vi "HEWH Find Exact Cutout Location.vi"(8 "error in (no error)":errorcluster, 10 "Upper Most Element":T6, 11 "UEF Calculated Values Input in":T1 {"Data Indexes"."15 sec after Draw Index" format="%#.2f"; "Data Indexes"."15 sec after Draw Timestamp" format="%#.2f"; "Data Indexes"."Test Start Timestamp" format="%.2f"; "Data Indexes"."Test End Timestamp" format="%.2f"; "Data Indexes"."T0 Timestamp" format="%.2f"; "Data Indexes"."Tsf Timestamp" format="%.2f"; "Data Indexes"."Tsu0 Timestamp" format="%.2f"; "Data Indexes"."Tmax1 Timestamp" format="%.2f"; "Data Indexes"."Draw Index Timestamp" format="%#.2f"; "Data Indexes"."Non-Draw Timestamp" format="%#.2f"; "Data Indexes"."Heating Timestamp" format="%#.2f"; "Data Indexes"."Start Energy (BTU-Gas)" format="%.6f"; "Data Indexes"."Start Watt Hours" format="%.6f"; "Static Data"."V - Volume of Wh (True)" format="%.5f"; "Static Data"."T-Ambinet Nominal (°F)" format="%.5f"; "Static Data"."T-Inlet Setpoint (°F)" format="%.5f"; "Static Data"."T-Wh Setpoint (°F)" format="%.5f"; "Sampled Data"."Qe (Wh)" format="%.5f"; "Sampled Data"."Tau stby2 (hr)" format="%.5f"; "Sampled Data"."Tastby2 (°F)" format="%.5f"; "Sampled Data"."Qf (BTU)" format="%.5f"; "Sampled Data"."Qe (BTU)" format="%.5f"; "Sampled Data"."Tmax1 (°F)" format="%.5f"; "Sampled Data"."T0 (°F)" format="%.5f"; "Sampled Data"."Qr (BTU)" format="%.5f"; "Sampled Data"."T 24(°F)" format="%.5f"; "Sampled Data"."T astby(°F)" format="%.5f"; "Sampled Data"."T tstby(°F)" format="%.5f"; "Sampled Data"."T su0(°F)" format="%.5f"; "Sampled Data"."T suf(°F)" format="%.5f"; "Sampled Data"."Tau stby_1 (hr)" format="%.5f"; "Sampled Data"."Qsuf (BTU)" format="%.5f"; "Sampled Data"."Qsu0 (BTU)" format="%.5f"; "Calculated Values"."Draw Bonus Volume (gal)" format="%.6f"; "Calculated Values"."Adjustment Factor" format="%.6f"; "Calculated Values"."T*avg_del(n-1)" format="%.6f"; "Calculated Values"."T*min(n-1)" format="%.6f"; "Calculated Values"."T*avg_del(n)" format="%.6f"; "Calculated Values"."Vn" format="%.6f"; "Calculated Values"."Qdm (BTU)" format="%.6f"; "Calculated Values"."QHWD (BTU)" format="%.6f"; "Calculated Values"."QHW (BTU)" format="%.6f"; "Calculated Values"."UEF" format="%.6f"; "Calculated Values"."QHW67 (BTU)" format="%.6f"; "Calculated Values"."Qda (BTU)" format="%.6f"; "Calculated Values"."Qd (BTU)" format="%.6f"; "Calculated Values"."Q (BTU)" format="%.6f"; "Calculated Values"."UA (BTU/(hr*F))" format="%.6f"; "Calculated Values"."Qhr (BTU/hr)" format="%.6f"; "Calculated Values"."Qstby (BTU)" format="%.6f"; "Calculated Values"."nu_r" format="%.6f"; "Calculated Values"."CpUEF (BTU/(lb*F))" format="%.6f"; "Calculated Values"."rho_nu (lb/gal)" format="%.6f"; "Calculated Values"."V1- Vol (Gal)" format="%.6f"; "Calculated Values"."M cluster mass removed (lb)" format="%.6f"; "Calculated Values"."Cp theoretical (BTU/(lbm °F))" format="%.6f"; "Calculated Values"."Tin1 - Mean Inlet 1st Cluster (°F)" format="%.6f"; "Calculated Values"."Tdel1-Mean Outlet 1st Cluster(°F)" format="%.6f"; "Calculated Values"."Cp 24 (BTU/(lb*F))" format="%.6f"; "Calculated Values"."Cp standby (BTU/(lb*F))" format="%.6f"; "Calculated Values"."Cp2 (BTU/(lb*F))" format="%.6f"; "Calculated Values"."Cp1 (BTU/(lb*F))" format="%.6f"; "Calculated Values"."rho 24 (lb/gal)" format="%.6f"; "Calculated Values"."rho standby (lb/gal)" format="%.6f"; "Calculated Values"."rho 2 (lb/gal)" format="%.6f"; "Calculated Values"."Density of cold water All (lbm/gal)" format="%#.3g"; "Calculated Values"."CpHW (BTU/(lbm °F))" format="%#.3g"; "Calculated Values"."Density of hot water All (lbm/gal)" format="%#.3g"; "Calculated Values"."Mass of water All (lbm)" format="%#.3f"}) -> (0 "error out":errorcluster, 2 "Cut Out Location":dbl, 3 "UEF Calculated Values Input in 2":T1 {"Data Indexes"."15 sec after Draw Index" format="%#.2f"; "Data Indexes"."15 sec after Draw Timestamp" format="%#.2f"; "Data Indexes"."Test Start Timestamp" format="%.2f"; "Data Indexes"."Test End Timestamp" format="%.2f"; "Data Indexes"."T0 Timestamp" format="%.2f"; "Data Indexes"."Tsf Timestamp" format="%.2f"; "Data Indexes"."Tsu0 Timestamp" format="%.2f"; "Data Indexes"."Tmax1 Timestamp" format="%.2f"; "Data Indexes"."Draw Index Timestamp" format="%#.2f"; "Data Indexes"."Non-Draw Timestamp" format="%#.2f"; "Data Indexes"."Heating Timestamp" format="%#.2f"; "Data Indexes"."Start Energy (BTU-Gas)" format="%.6f"; "Data Indexes"."Start Watt Hours" format="%.6f"; "Static Data"."V - Volume of Wh (True)" format="%.5f"; "Static Data"."T-Ambinet Nominal (°F)" format="%.5f"; "Static Data"."T-Inlet Setpoint (°F)" format="%.5f"; "Static Data"."T-Wh Setpoint (°F)" format="%.5f"; "Sampled Data"."Qe (Wh)" format="%.5f"; "Sampled Data"."Tau stby2 (hr)" format="%.5f"; "Sampled Data"."Tastby2 (°F)" format="%.5f"; "Sampled Data"."Qf (BTU)" format="%.5f"; "Sampled Data"."Qe (BTU)" format="%.5f"; "Sampled Data"."Tmax1 (°F)" format="%.5f"; "Sampled Data"."T0 (°F)" format="%.5f"; "Sampled Data"."Qr (BTU)" format="%.5f"; "Sampled Data"."T 24(°F)" format="%.5f"; "Sampled Data"."T astby(°F)" format="%.5f"; "Sampled Data"."T tstby(°F)" format="%.5f"; "Sampled Data"."T su0(°F)" format="%.5f"; "Sampled Data"."T suf(°F)" format="%.5f"; "Sampled Data"."Tau stby_1 (hr)" format="%.5f"; "Sampled Data"."Qsuf (BTU)" format="%.5f"; "Sampled Data"."Qsu0 (BTU)" format="%.5f"; "Calculated Values"."Draw Bonus Volume (gal)" format="%.6f"; "Calculated Values"."Adjustment Factor" format="%.6f"; "Calculated Values"."T*avg_del(n-1)" format="%.6f"; "Calculated Values"."T*min(n-1)" format="%.6f"; "Calculated Values"."T*avg_del(n)" format="%.6f"; "Calculated Values"."Vn" format="%.6f"; "Calculated Values"."Qdm (BTU)" format="%.6f"; "Calculated Values"."QHWD (BTU)" format="%.6f"; "Calculated Values"."QHW (BTU)" format="%.6f"; "Calculated Values"."UEF" format="%.6f"; "Calculated Values"."QHW67 (BTU)" format="%.6f"; "Calculated Values"."Qda (BTU)" format="%.6f"; "Calculated Values"."Qd (BTU)" format="%.6f"; "Calculated Values"."Q (BTU)" format="%.6f"; "Calculated Values"."UA (BTU/(hr*F))" format="%.6f"; "Calculated Values"."Qhr (BTU/hr)" format="%.6f"; "Calculated Values"."Qstby (BTU)" format="%.6f"; "Calculated Values"."nu_r" format="%.6f"; "Calculated Values"."CpUEF (BTU/(lb*F))" format="%.6f"; "Calculated Values"."rho_nu (lb/gal)" format="%.6f"; "Calculated Values"."V1- Vol (Gal)" format="%.6f"; "Calculated Values"."M cluster mass removed (lb)" format="%.6f"; "Calculated Values"."Cp theoretical (BTU/(lbm °F))" format="%.6f"; "Calculated Values"."Tin1 - Mean Inlet 1st Cluster (°F)" format="%.6f"; "Calculated Values"."Tdel1-Mean Outlet 1st Cluster(°F)" format="%.6f"; "Calculated Values"."Cp 24 (BTU/(lb*F))" format="%.6f"; "Calculated Values"."Cp standby (BTU/(lb*F))" format="%.6f"; "Calculated Values"."Cp2 (BTU/(lb*F))" format="%.6f"; "Calculated Values"."Cp1 (BTU/(lb*F))" format="%.6f"; "Calculated Values"."rho 24 (lb/gal)" format="%.6f"; "Calculated Values"."rho standby (lb/gal)" format="%.6f"; "Calculated Values"."rho 2 (lb/gal)" format="%.6f"; "Calculated Values"."Density of cold water All (lbm/gal)" format="%#.3g"; "Calculated Values"."CpHW (BTU/(lbm °F))" format="%#.3g"; "Calculated Values"."Density of hot water All (lbm/gal)" format="%#.3g"; "Calculated Values"."Mass of water All (lbm)" format="%#.3f"})   [LabVIEW 2023]
uses:
  Type Definitions/UEF Constants.ctl
  Type Definitions/HEWH Draw Stats.ctl
  Type Definitions/HEWH FHR Draw Type.ctl
  Type Definitions/FHR Bins.ctl
  Type Definitions/HEWH Meter Type.ctl
  Type Definitions/Upper Most Element.ctl
panel:
  # "FHR"
  # "FHR"
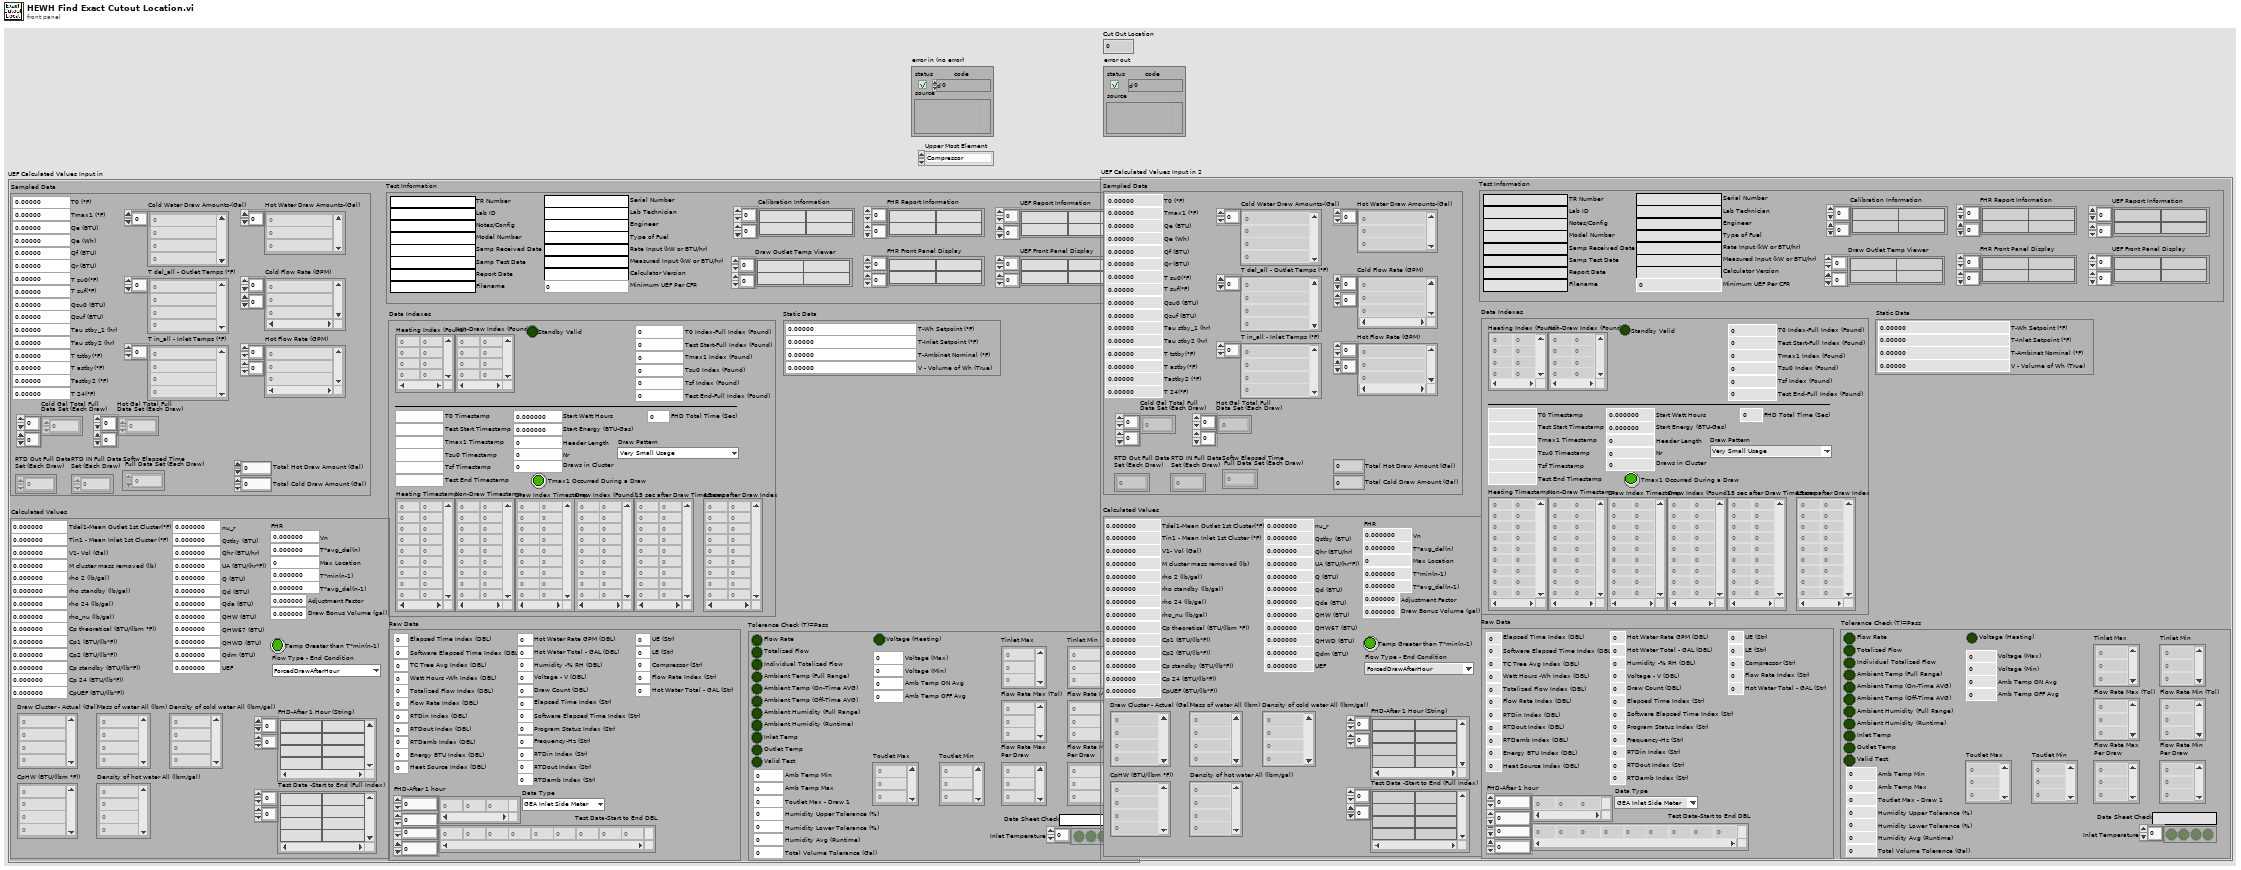
[diagram p1: front panel]
types:
  T1 = typedef "UEF Constants.ctl" = cluster{"Calculated Values":T2, "Sampled Data":cluster{"Cold Water Draw Amounts-(Gal)":dbl[], "T del_all - Outlet Temps (°F)":dbl[], "T in_all - Inlet Temps (°F)":dbl[], "Qsu0 (BTU)":dbl, "Qsuf (BTU)":dbl, "Tau stby_1 (hr)":dbl, "T suf(°F)":dbl, "T su0(°F)":dbl, "T tstby(°F)":dbl, "T astby(°F)":dbl, "T 24(°F)":dbl, "Qr (BTU)":dbl, "T0 (°F)":dbl, "Tmax1 (°F)":dbl, "Qe (BTU)":dbl, "Qf (BTU)":dbl, "Tastby2 (°F)":dbl, "RTD Out Full Data\nSet (Each Draw)":dbl[][], "RTD IN Full Data\nSet (Each Draw)":dbl[][], "Tau stby2 (hr)":dbl, "Hot Water Draw Amounts-(Gal)":dbl[], "Cold Flow Rate (GPM)":dbl[][], "Hot Flow Rate (GPM)":dbl[][], "Softw Elapsed Time\n Full Data Set (Each Draw)":dbl[][], "Cold Gal Total Full\nData Set (Each Draw)":dbl[][], "Total Hot Draw Amount (Gal) ":dbl, "Total Cold Draw Amount (Gal)":dbl, "Qe (Wh)":dbl, "Hot Gal Total Full\nData Set (Each Draw)":dbl[][]}, "Static Data":cluster{"T-Wh Setpoint (°F)":dbl, "T-Inlet Setpoint (°F)":dbl, "T-Ambinet Nominal (°F)":dbl, "V - Volume of Wh (True)":dbl}, "Data Indexes":cluster{"Test Start-Full Index (Found)":i32, "Header Length":i32, "Draw Index (Found)":i32[][], "Nr":i32, "Start Watt Hours":dbl, "Tsu0 Index (Found)":i32, "Tsf Index (Found)":i32, "Start Energy (BTU-Gas)":dbl, "Draws in Cluster":i32, "T0 Index-Full Index (Found)":i32, "Non-Draw Index (Found)":i32[][], "Tmax1 Index (Found)":i32, "Test End-Full Index (Found)":i32, "Heating Index (Found)":i32[][], "Heating Timestamp":dbl[][], "Non-Draw Timestamp":dbl[][], "Draw Index Timestamp":dbl[][], "Tmax1 Timestamp":dbl, "Tsu0 Timestamp":dbl, "Tsf Timestamp":dbl, "T0 Timestamp":dbl, "Test End Timestamp":dbl, "Test Start Timestamp":dbl, "15 sec after Draw Timestamp":dbl[][], "15 sec after Draw Index":dbl[][], "Tmax1 Occurred During a Draw":bool, "FHD Total Time (Sec)":dbl, "Draw Pattern":T4, "Standby Valid":bool}, "Raw Data":cluster{"Elapsed Time Index (DBL)":i32, "Software Elapsed Time Index (DBL)":i32, "TC Tree Avg Index (DBL)":i32, "Watt Hours -Wh Index (DBL)":i32, "Energy BTU Index (DBL)":i32, "Totalized Flow Index (DBL)":i32, "Flow Rate Index (DBL)":i32, "Program Status Index (Str)":i32, "RTDin Index (DBL)":i32, "RTDout Index (DBL)":i32, "RTDamb Index (DBL)":i32, "Test Data-Start to End DBL":dbl[][], "Data Type":T5, "Heat Source Index (DBL)":i32, "Hot Water Rate GPM (DBL)":i32, "Hot Water Total - GAL (DBL)":i32, "FHD-After 1 hour":dbl[][], "Humidity -% RH (DBL)":i32, "Voltage - V (DBL)":i32, "Draw Count (DBL)":i32, "Elapsed Time Index (Str)":i32, "Software Elapsed Time Index (Str)":i32, "Frequency-Hz (Str)":i32, "RTDin Index (Str)":i32, "RTDout Index (Str)":i32, "RTDamb Index (Str)":i32, "UE (Str)":i32, "LE (Str)":i32, "Compressor (Str)":i32, "Flow Rate Index (Str)":i32, "Hot Water Total - GAL (Str)":i32}, "Tolerance Check (T)=Pass":cluster{"Flow Rate":bool, "Totalized Flow":bool, "Ambient Temp (Full Range)":bool, "Ambient Humidity (Full Range)":bool, "Inlet Temp":bool, "Outlet Temp":bool, "Valid Test":bool, "Individual Totalized Flow":bool, "Data Sheet Check":string, "Inlet Temperature":bool[], "Tinlet Max":dbl[], "Tinlet Min":dbl[], "Flow Rate Max (Tol)":dbl[], "Flow Rate Min (Tol)":dbl[], "Amb Temp Max":dbl, "Amb Temp Min":dbl, "Toutlet Max - Draw 1":dbl, "Humidity Upper Tolerance (%)":dbl, "Total Volume Tolerance (Gal)":dbl, "Humidity Lower Tolerance (%)":dbl, "Flow Rate Max\nPer Draw":dbl[], "Flow Rate Min\nPer Draw":dbl[], "Ambient Humidity (Runtime)":bool, "Humidity Avg (Runtime)":dbl, "Ambient Temp (On-Time AVG)":bool, "Ambient Temp (Off-Time AVG)":bool, "Amb Temp OFF Avg":dbl, "Amb Temp ON Avg":dbl, "Voltage (Heating)":bool, "Voltage (Min)":dbl, "Voltage (Max)":dbl, "Toutlet Max":dbl[], "Toutlet Min":dbl[]}, "Test Information":cluster{"TR Number":string, "Lab ID":string, "Notes/Config":string, "Model Number":string, "Serial Number":string, "Lab Technician":string, "Engineer":string, "Type of Fuel":string, "Samp Received Date":string, "Samp Test Date":string, "Report Date":string, "Rate Input (kW or BTU/hr)":string, "Measured Input (kW or BTU/hr)":string, "Filename":string, "Calibration Information":string[][], "Calculator Version":string, "Minimum UEF Per CFR":dbl, "UEF Report Information":string[][], "FHR Report Information":string[][], "FHR Front Panel Display":string[][], "UEF Front Panel Display":string[][], "Draw Outlet Temp Viewer":string[][]}}
  T2 = typedef "HEWH Draw Stats.ctl" = cluster{"Draw Cluster - Actual (Gal)":dbl[], "Mass of water All (lbm)":dbl[], "Density of hot water All (lbm/gal)":dbl[], "CpHW (BTU/(lbm °F))":dbl[], "rho 2 (lb/gal)":dbl, "rho standby (lb/gal)":dbl, "rho 24 (lb/gal)":dbl, "Cp1 (BTU/(lb*F))":dbl, "Cp2 (BTU/(lb*F))":dbl, "Cp standby (BTU/(lb*F))":dbl, "Cp 24 (BTU/(lb*F))":dbl, "nu_r":dbl, "Qstby (BTU)":dbl, "Qhr (BTU/hr)":dbl, "UA (BTU/(hr*F))":dbl, "Q (BTU)":dbl, "Qd (BTU)":dbl, "Qda (BTU)":dbl, "QHW67 (BTU)":dbl, "UEF":dbl, "Tdel1-Mean Outlet 1st Cluster(°F)":dbl, "Tin1 - Mean Inlet 1st Cluster (°F)":dbl, "Cp theoretical (BTU/(lbm °F))":dbl, "M cluster mass removed (lb)":dbl, "V1- Vol (Gal)":dbl, "Test Data -Start to End (Full Index)":string[][], "rho_nu (lb/gal)":dbl, "Density of cold water All (lbm/gal)":dbl[], "CpUEF (BTU/(lb*F))":dbl, "QHW (BTU)":dbl, "QHWD (BTU)":dbl, "Qdm (BTU)":dbl, "FHD-After 1 Hour (String)":string[][], "Vn":dbl, "T*avg_del(n)":dbl, "Max Location":i32, "T*min(n-1)":dbl, "T*avg_del(n-1)":dbl, "Temp Greater than T*min(n-1)":bool, "Adjustment Factor":dbl, "Draw Bonus Volume (gal)":dbl, "Flow Type - End Condition":T3}
  T3 = typedef "HEWH FHR Draw Type.ctl" = enum16{"ForcedDrawAfterHour", "HeatingCutoffBeforeHour"}
  T4 = typedef "FHR Bins.ctl" = enum16{"Very Small Usage", "Low Usage", "Medium Usage", "High Usage", "Undefined"}
  T5 = typedef "HEWH Meter Type.ctl" = enum16{"GEA Inlet Side Meter", "GEA Outlet Side Meter", "CSA Inlet Side Meter"}
  T6 = typedef "Upper Most Element.ctl" = enum16{"Compressor", "Lower Element", "Upper Element"}
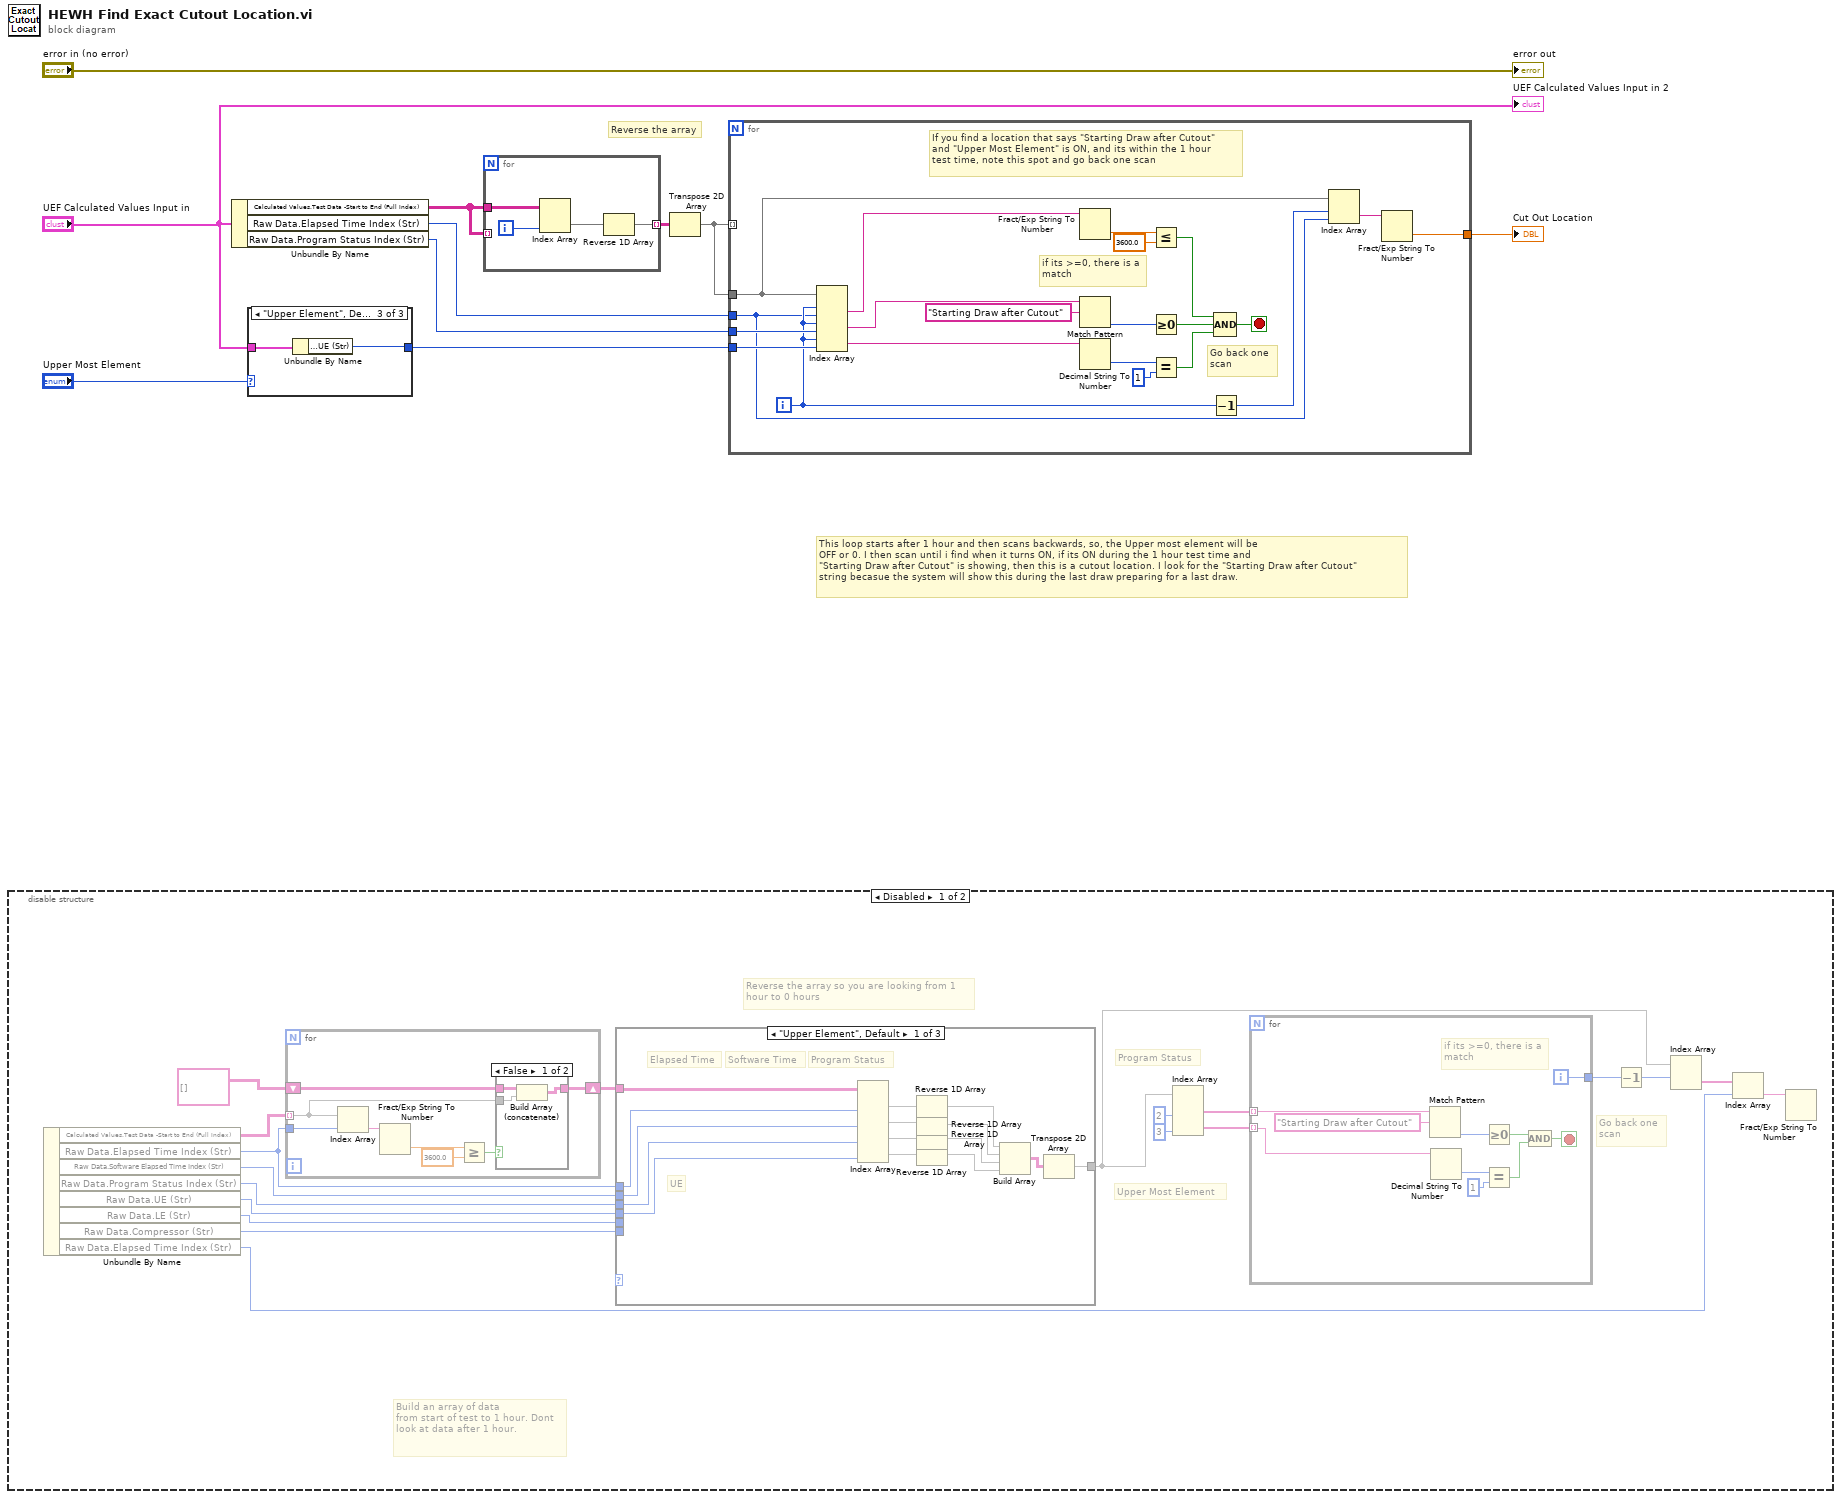
[diagram p0: block diagram]
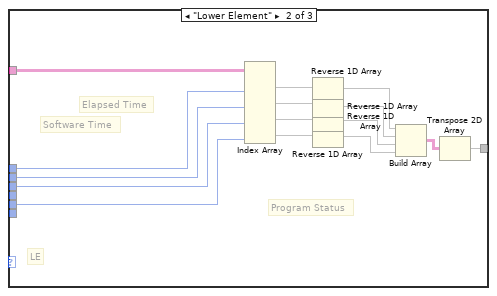
[diagram p2: hidden frame]
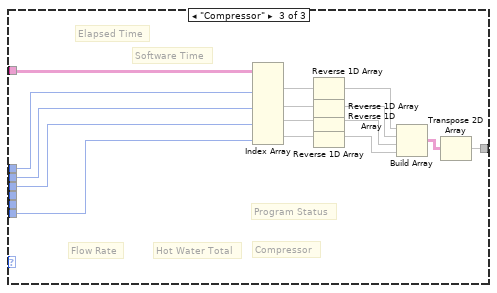
[diagram p3: hidden frame]
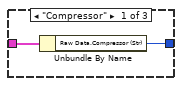
[diagram p6: hidden frame]
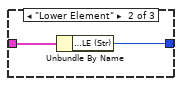
[diagram p7: hidden frame]
diagram:
  # "This loop starts after 1 hour and then scans backwards, so, the Upper most element will be \nOFF or 0. I then scan until i find when it turns ON, if its ON during the 1 hour test time and\n\"Starting Draw after Cutout\" is showing, then this is a cutout location. I look for the \"Starting Draw after Cutout\"\nstring becasue the system will show this during the last draw preparing for a last draw."
  # "Reverse the array"
  n1 = disable-structure shown="Disabled" {
    frame Disabled {
      # "Reverse the array so you are looking from 1\nhour to 0 hours"
      # "Go back one\nscan"
      # "Upper Most Element"
      # "Program Status"
      # "Build an array of data\nfrom start of test to 1 hour. Dont look at data after 1 hour."
      n2 = Unbundle By Name() -> ("Calculated Values.Test Data -Start to End (Full Index)"=w11:string[][], "Raw Data.Elapsed Time Index (Str)"=w14:i32, "Raw Data.Software Elapsed Time Index (Str)"=w20:i32, "Raw Data.Program Status Index (Str)"=w19:i32, "Raw Data.UE (Str)"=w18:i32, "Raw Data.LE (Str)"=w17:i32, "Raw Data.Compressor (Str)"=w16:i32, "Raw Data.Elapsed Time Index (Str)"=w13:i32)  [unwired: 1 in]
      n3 = for {
        tunnel: w11 -> [w86] mode=indexing
        shift-right: [w91] -> w15
        shift-left: string[][] [] -> [w92]
        tunnel: w14 -> [w85]
        n4 = Index Array(array=w86, index=w85) -> (element=w90:string)
        n5 = Fract/Exp String To Number(string=w90) -> (number=w89:dbl)  [unwired: 3 in, 1 out]
        n6 = Greater Or Equal?(x=w89, y=3600.0) -> (x >= y?=w87:bool)
        n7 = case shown="False" w87 {
          tunnel: w92 -> [w95 w96]
          tunnel: [w94 w96] -> w91
          tunnel: w86 -> [w93 _]
          frame False {
            n8 = Build Array (concatenate)(w95, w93) -> (w94:string[][])
          }
          frame True {
          }
        }
      }
      n9 = case shown="\"Upper Element\", Default" {
        selector: _ -> [_ _ _]
        tunnel: w15 -> [w53 w69 w84]
        tunnel: [w52 w59 w74] -> w26
        tunnel: w14 -> [w43 w58 w73]
        tunnel: w20 -> [w42 w57 w72]
        tunnel: w19 -> [w41 w56 w71]
        tunnel: w18 -> [w40 _ _]
        tunnel: w17 -> [_ w55 _]
        tunnel: w16 -> [_ _ w70]
        frame "Upper Element", Default {
          # "UE"
          # "Program Status"
          # "Software Time"
          # "Elapsed Time"
          n10 = Index Array(array=w53, index (col) #1=w43, index (col) #2=w42, index (col) #3=w41, index (col) #4=w40) -> (element #1=w51:string[], element #2=w49:string[], element #3=w47:string[], element #4=w45:string[])  [unwired: 4 in]
          n11 = Reverse 1D Array(array=w51) -> (reversed array=w50:string[])
          n12 = Reverse 1D Array(array=w49) -> (reversed array=w48:string[])
          n13 = Reverse 1D Array(array=w47) -> (reversed array=w46:string[])
          n14 = Reverse 1D Array(array=w45) -> (reversed array=w44:string[])
          n15 = Build Array(w50, w48, w46, w44) -> (w54:string[][])
          n16 = Transpose 2D Array(2D array=w54) -> (transposed array=w52:string[][])
        }
        frame "Lower Element" {
          # "LE"
          # "Program Status"
          # "Software Time"
          # "Elapsed Time"
          n17 = Index Array(array=w69, index (col) #1=w58, index (col) #2=w57, index (col) #3=w56, index (col) #4=w55) -> (element #1=w63:string[], element #2=w62:string[], element #3=w61:string[], element #4=w60:string[])  [unwired: 4 in]
          n18 = Reverse 1D Array(array=w63) -> (reversed array=w67:string[])
          n19 = Reverse 1D Array(array=w62) -> (reversed array=w66:string[])
          n20 = Reverse 1D Array(array=w61) -> (reversed array=w65:string[])
          n21 = Reverse 1D Array(array=w60) -> (reversed array=w64:string[])
          n22 = Build Array(w67, w66, w65, w64) -> (w68:string[][])
          n23 = Transpose 2D Array(2D array=w68) -> (transposed array=w59:string[][])
        }
        frame "Compressor" {
          # "Hot Water Total"
          # "Program Status"
          # "Flow Rate"
          # "Compressor"
          # "Software Time"
          # "Elapsed Time"
          n24 = Index Array(array=w84, index (col) #1=w73, index (col) #2=w72, index (col) #3=w71, index (col) #4=w70) -> (element #1=w78:string[], element #2=w77:string[], element #3=w76:string[], element #4=w75:string[])  [unwired: 4 in]
          n25 = Reverse 1D Array(array=w78) -> (reversed array=w82:string[])
          n26 = Reverse 1D Array(array=w77) -> (reversed array=w81:string[])
          n27 = Reverse 1D Array(array=w76) -> (reversed array=w80:string[])
          n28 = Reverse 1D Array(array=w75) -> (reversed array=w79:string[])
          n29 = Build Array(w82, w81, w80, w79) -> (w83:string[][])
          n30 = Transpose 2D Array(2D array=w83) -> (transposed array=w74:string[][])
        }
      }
      n31 = Index Array(array=w26, index (col) #1=2 ("disabled index (col)"), index (col) #2=3 ("index (col)")) -> (element #1=w12:string[], element #2=w24:string[])  [unwired: 2 in]
      n32 = for {
        tunnel: w12 -> [w39] mode=indexing
        tunnel: w24 -> [w37] mode=indexing
        tunnel: [w32] -> w25
        i -> [w32]
        stop <- w33 stop-if-true
        # "if its >=0, there is a \nmatch"
        n33 = Match Pattern(string=w39, regular expression="Starting Draw after Cutout") -> (offset past match=w31:i32)  [unwired: 1 in, 3 out]
        n34 = Decimal String To Number(string=w37) -> (number=w36:i32)  [unwired: 2 in, 1 out]
        n35 = Greater Or Equal To 0?(x=w31) -> (x >= 0?=w30:bool)
        n36 = Equal?(x=w36, y=1) -> (x = y?=w34:bool)
        n37 = Compound Arithmetic op=AND(w30, w34) -> (w33:bool)
      }
      n38 = Decrement(x=w25) -> (x-1=w27:i32)
      n39 = Index Array(array=w26, index (row)=w27) -> (element=w28:string[])  [unwired: 1 in]
      n40 = Index Array(array=w28, index=w13) -> (element=w29:string)
      n41 = Fract/Exp String To Number(string=w29) -> ()  [unwired: 3 in, 2 out]
    }
    frame Enabled {
    }
  }
  n42 = Unbundle By Name("UEF Calculated Values Input in") -> ("Calculated Values.Test Data -Start to End (Full Index)"=w2:string[][], "Raw Data.Elapsed Time Index (Str)"=w8:i32, "Raw Data.Program Status Index (Str)"=w7:i32)
  n43 = case shown="\"Upper Element\", Default" "Upper Most Element" {
    tunnel: "UEF Calculated Values Input in" -> [w98 w100 w102]
    tunnel: [w97 w99 w101] -> w4
    frame "Compressor" {
      n44 = Unbundle By Name(w98) -> ("Raw Data.Compressor (Str)"=w97:i32)
    }
    frame "Lower Element" {
      n45 = Unbundle By Name(w100) -> ("Raw Data.LE (Str)"=w99:i32)
    }
    frame "Upper Element", Default {
      n46 = Unbundle By Name(w102) -> ("Raw Data.UE (Str)"=w101:i32)
    }
  }
  n47 = for {
    tunnel: w2 -> [w106]
    tunnel: w2 -> [_] mode=indexing
    tunnel: [w103] -> w9 mode=indexing
    i -> [w105]
    n48 = Index Array(array=w106, index (col)=w105) -> (element=w104:string[])  [unwired: 1 in]
    n49 = Reverse 1D Array(array=w104) -> (reversed array=w103:string[])
  }
  n50 = Transpose 2D Array(2D array=w9) -> (transposed array=w3:string[][])
  n51 = for {
    tunnel: w3 -> [_] mode=indexing
    tunnel: w8 -> [w110]
    tunnel: w7 -> [w127]
    tunnel: w4 -> [w126]
    tunnel: w3 -> [w112]
    tunnel: [w108] -> w1
    i -> [w113]
    stop <- w107 stop-if-true
    # "Go back one\nscan"
    # "If you find a location that says \"Starting Draw after Cutout\"\nand \"Upper Most Element\" is ON, and its within the 1 hour\ntest time, note this spot and go back one scan"
    # "if its >=0, there is a \nmatch"
    n52 = Index Array(array=w112, index (row) #1=w113, index (col) #1=w110, index (row) #2=w113, index (col) #2=w127, index (row) #3=w113, index (col) #3=w126) -> (element #1=w115:string, element #2=w119:string, element #3=w118:string)
    n53 = Fract/Exp String To Number(string=w115) -> (number=w116:dbl)  [unwired: 3 in, 1 out]
    n54 = Match Pattern(string=w119, regular expression="Starting Draw after Cutout") -> (offset past match=w123:i32)  [unwired: 1 in, 3 out]
    n55 = Decimal String To Number(string=w118) -> (number=w125:i32)  [unwired: 2 in, 1 out]
    n56 = Less Or Equal?(x=w116, y=3600.0) -> (x <= y?=w114:bool)
    n57 = Greater Or Equal To 0?(x=w123) -> (x >= 0?=w122:bool)
    n58 = Equal?(x=w125, y=1) -> (x = y?=w124:bool)
    n59 = Decrement(x=w113) -> (x-1=w111:i32)
    n60 = Compound Arithmetic op=AND(w114, w122, w124) -> (w107:bool)
    n61 = Index Array(array=w112, index (row)=w111, index (col)=w110) -> (element=w109:string)
    n62 = Fract/Exp String To Number(string=w109) -> (number=w108:dbl)  [unwired: 3 in, 1 out]
  }
  "Cut Out Location" <- w1
  "error out" <- "error in (no error)"
  "UEF Calculated Values Input in 2" <- "UEF Calculated Values Input in"
